vi "lifecam.vi"() -> ()   [LabVIEW 2015]
uses:
  <vilib>/userdefined/High Color/IMAQdx.ctl
  <vilib>/vision/driver/NI_Vision_Acquisition_Software.lvlib
panel:
  out "Image":T1(plugin-control)
  in  "Session In":T2
  in  "stop":bool
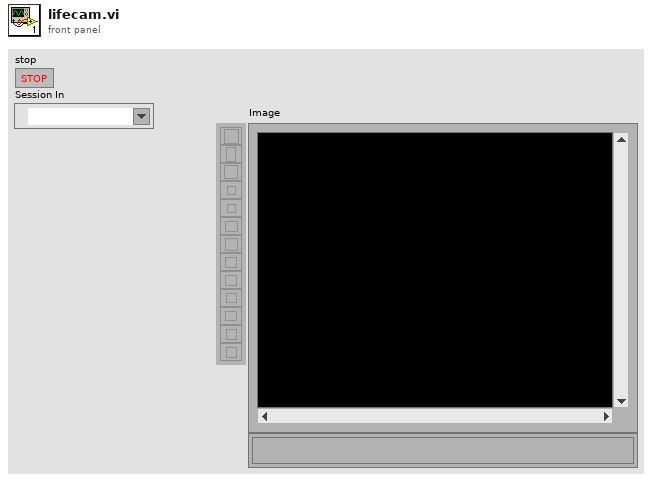
[diagram p1: front panel]
types:
  T1 = typedef "IMAQ Image.ctl" = refnum<image>
  T2 = typedef "IMAQdx.ctl" = refnum<k21>
  T3 = typedef "Image Type" = u32
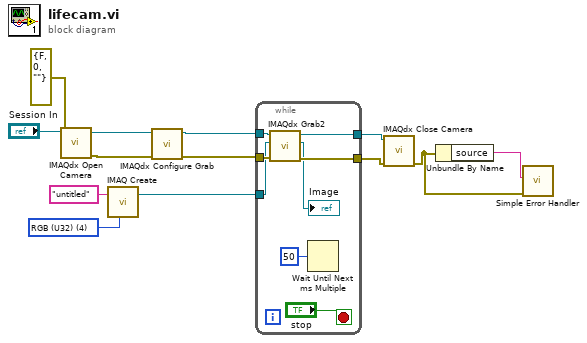
[diagram p0: block diagram]
diagram:
  w8 = T3 4 items=["Grayscale (U8)", "Grayscale (I16)", "Grayscale (SGL)", "Complex (CSG)", "RGB (U32)", "HSL (U32)", "RGB (U64)", "Grayscale (U16)"] ("Image Type")
  n1 = call <vilib>:"IMAQdx Open Camera.vi"("error in"=errorcluster {"status"=FALSE, "code"=0, "source"=""}, "Session In"="Session In") -> ("error out"=w2:errorcluster, "Session Out"=w1:T2)  [unwired: 8 in]
  n2 = call "IMAQ Create"("Image Name"="untitled", "Image Type"=w8) -> ("New Image"=w7:T1)  [unwired: 3 in, 1 out]
  n3 = call <vilib>:"IMAQdx Configure Grab.vi"("error in"=w2, "Session In"=w1) -> ("error out"=w3:errorcluster, "Session Out"=w4:T2)  [unwired: 8 in]
  n4 = while {
    tunnel: w4 -> [w20]
    tunnel: w3 -> [w19]
    tunnel: [w18] -> w11
    tunnel: [w17] -> w10
    tunnel: w7 -> [w16]
    stop <- "stop" stop-if-true
    n5 = call <vilib>:"IMAQdx Grab2.vi"("error in"=w19, "Image In"=w16, "Session In"=w20) -> ("error out"=w17:errorcluster, "Image Out"=→"Image":T1, "Session Out"=w18:T2)  [unwired: 5 in, 1 out]
    n6 = Wait Until Next ms Multiple(millisecond multiple=u32 50) -> ()  [unwired: 1 out]
  }
  n7 = call <vilib>:"IMAQdx Close Camera.vi"("error in"=w10, "Session In"=w11) -> ("error out"=w6:errorcluster)  [unwired: 9 in]
  n8 = Unbundle By Name(w6) -> ("source"=w5:string)
  n9 = call <vilib>:"Simple Error Handler.vi"("error source (\" \")"=w5, "error in (no error)"=w6) -> ()  [unwired: 3 in, 5 out]
